vi "generateSimulatedData.vi"(8 "error in (no error)":errorcluster, 11 "ILCSim1 in":refnum<class "ILCSim1.lvclass">) -> (0 "error out":errorcluster, 2 "stringRead":string, 3 "ILCSim1 out":refnum<class "ILCSim1.lvclass">)   [LabVIEW 2013, in "ILCSim1.lvclass"]
uses:
  ILCSim1.lvclass
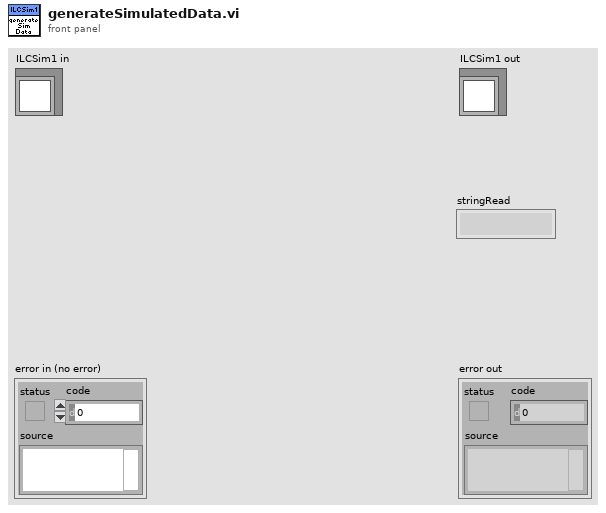
[diagram p1: front panel]
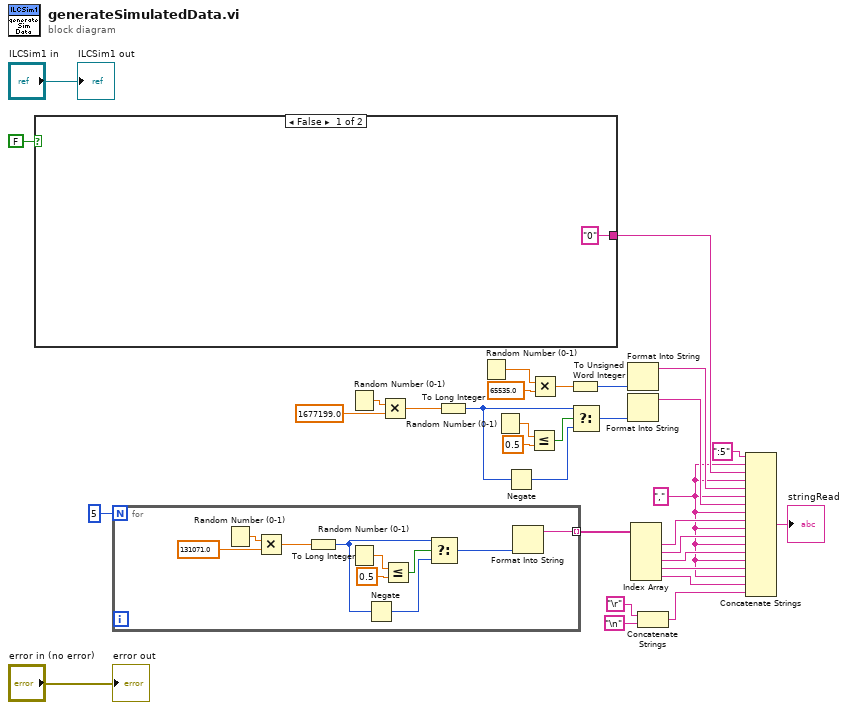
[diagram p0: block diagram]
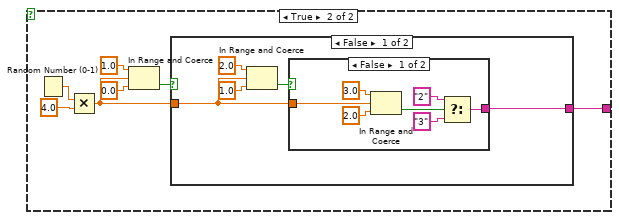
[diagram p2: hidden frame]
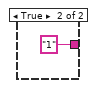
[diagram p3: hidden frame]
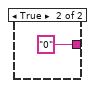
[diagram p4: hidden frame]
diagram:
  w6 = "," ("string")
  n1 = case shown="False" FALSE {
    tunnel: ["0" ("string") w35] -> w31
    frame False {
    }
    frame True {
      n2 = Random Number (0-1)() -> (number: 0 to 1=w40:dbl)
      n3 = Multiply(x=w40, y=4.0) -> (x*y=w34:dbl)
      n4 = In Range and Coerce(upper limit=1.0, x=w34, lower limit=0.0) -> (In Range?=w36:bool)  [unwired: 1 out]
      n5 = case shown="False" w36 {
        tunnel: [w42 "0" ("string")] -> w35
        tunnel: w34 -> [w41 _]
        frame False {
          n6 = In Range and Coerce(upper limit=2.0, x=w41, lower limit=1.0) -> (In Range?=w43:bool)  [unwired: 1 out]
          n7 = case shown="False" w43 {
            tunnel: [w47 "1" ("string")] -> w42
            tunnel: w41 -> [w46 _]
            frame False {
              n8 = In Range and Coerce(upper limit=3.0, x=w46, lower limit=2.0) -> (In Range?=w50:bool)  [unwired: 1 out]
              n9 = Select(t="2" ("string"), s=w50, f="3" ("string")) -> (s? t:f=w47:string)
            }
            frame True {
            }
          }
        }
        frame True {
        }
      }
    }
  }
  n10 = for {
    N: 5 -> [_]
    tunnel: [w55] -> w11 mode=indexing
    n11 = Random Number (0-1)() -> (number: 0 to 1=w56:dbl)
    n12 = Multiply(x=w56, y=131071.0) -> (x*y=w60:dbl)
    n13 = To Long Integer(number=w60) -> (32bit integer=w61:i32)
    n14 = Random Number (0-1)() -> (number: 0 to 1=w58:dbl)
    n15 = Negate(x=w61) -> (-x=w63:i32)
    n16 = Less Or Equal?(x=w58, y=0.5) -> (x <= y?=w62:bool)
    n17 = Select(t=w61, s=w62, f=w63) -> (s? t:f=w64:i32)
    n18 = Format Into String(w64) -> (resulting string=w55:string)  [unwired: 3 in, 1 out]
  }
  n19 = Random Number (0-1)() -> (number: 0 to 1=w25:dbl)
  n20 = Multiply(x=w25, y=1677199.0) -> (x*y=w21:dbl)
  n21 = To Long Integer(number=w21) -> (32bit integer=w20:i32)
  n22 = Random Number (0-1)() -> (number: 0 to 1=w29:dbl)
  n23 = Random Number (0-1)() -> (number: 0 to 1=w23:dbl)
  n24 = Negate(x=w20) -> (-x=w18:i32)
  n25 = Less Or Equal?(x=w23, y=0.5) -> (x <= y?=w19:bool)
  n26 = Multiply(x=w29, y=65535.0) -> (x*y=w28:dbl)
  n27 = To Unsigned Word Integer(number=w28) -> (unsigned 16bit integer=w27:u16)
  n28 = Select(t=w20, s=w19, f=w18) -> (s? t:f=w17:i32)
  n29 = Format Into String(w27) -> (resulting string=w26:string)  [unwired: 3 in, 1 out]
  n30 = Format Into String(w17) -> (resulting string=w16:string)  [unwired: 3 in, 1 out]
  n31 = Index Array(array=w11) -> (element #1=w10:string, element #2=w9:string, element #3=w8:string, element #4=w7:string, element #5=w5:string)  [unwired: 5 in]
  n32 = Concatenate Strings("\r", "\n") -> (w13:string)
  n33 = Concatenate Strings(":5" ("string"), w6, w31, w6, w26, w6, w16, w6, w10, w6, w9, w6, w8, w6, w7, w6, w5, w13) -> (→"stringRead":string)
  "error out" <- "error in (no error)"
  "ILCSim1 out" <- "ILCSim1 in"
